vi "zmiana czcionki w string.vi"() -> ()   [LabVIEW 2013]
panel:
  in  "stop":bool
  in  "Boolean":bool
  in  "Text.Font:Name":string
  out "String 2":string
  out "*(type *) &x":u8
  in  "String":string
  out "appended array":string[][](array[string])
  # "liczenie"
  # "0-11"
  # "12-23"
  # "24-35"
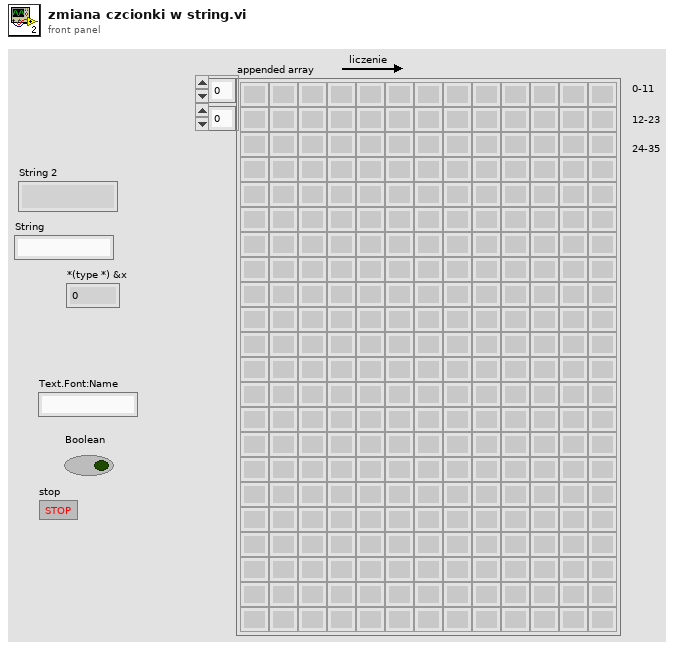
[diagram p1: front panel]
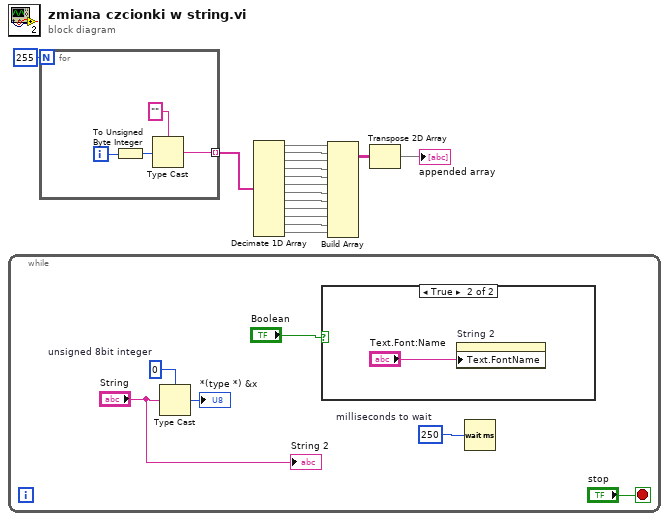
[diagram p0: block diagram]
diagram:
  n1 = while {
    stop <- "stop" stop-if-true
    w18 = u32 250  # milliseconds to wait
    w22 = u8 0  # unsigned 8bit integer
    n2 = Type Cast(type=w22, x="String") -> (*(type *) &x=→"*(type *) &x":u8)
    n3 = case shown="True" "Boolean" {
      frame False {
      }
      frame True {
        n4 = property on="String 2" class="Str"("Text.FontName"="Text.Font:Name") -> ()  [unwired: 2 in, 2 out]
      }
    }
    n5 = Wait (ms)(milliseconds to wait=w18) -> ()  [unwired: 1 out]
    "String 2" <- "String"
  }
  n6 = for {
    N: 255 -> [_]
    tunnel: [w24] -> w15 mode=indexing
    i -> [w27]
    n7 = To Unsigned Byte Integer(number=w27) -> (unsigned 8bit integer=w26:u8)
    n8 = Type Cast(type="", x=w26) -> (*(type *) &x=w24:string)
  }
  n9 = Decimate 1D Array(w15) -> (w14:string[], w13:string[], w12:string[], w11:string[], w8:string[], w7:string[], w6:string[], w5:string[], w4:string[], w3:string[], w2:string[], w1:string[])
  n10 = Build Array(w14, w13, w12, w11, w8, w7, w6, w5, w4, w3, w2, w1) -> (w10:string[][])
  n11 = Transpose 2D Array(2D array=w10) -> (transposed array=→"appended array":string[][])
